vi "run pivot files.vi"() -> ()   [LabVIEW 2013]
uses:
  <vilib>/Utility/file.llb/Read From Spreadsheet File (DBL).vi
panel:
  in  "Tab Control":enum32{"Load Files", "Run"}(tab)
  in  "file path":path=path "C:/Program Files/Labview/user.lib/ROSforLV_0.1/Devices/Baxter/NIST2/Circles (Nick)"
  out "filenames":string[](array[string])=["Pivot a25 s15 r370 n0_0.csv", "Pivot a25 s20 r370 n0_0.csv", "Pivot a25 s20 r370 n0_5.csv", "Pivot a25 s20 r370 n1_0.csv", "Pivot a25 s20 r370 n1_5.csv", "Pivot a25 s20 r370 n2_0.csv", "Pivot a25 s20 r370 n2_5.csv", "Pivot a25 s20 r370 n3_0.csv", "Pivot a25 s20 r370 n3_5.csv", "Pivot a25 s20 r370 n4_0.csv", "Pivot a25 s25 r370 n0_0.csv", "Pivot a25 s30 r370 n0_0.csv", "Pivot a25 s35 r370 n0_0.csv"]
  out "Loop":i32
  out "of":i32
  in  "Abort":bool
  in  "Cycles":i32
  out "Status":string[](array[string])=["Initializing"]
  # "Execute this tab first to see the avialable files.\nThen remove the undesired trajectories before running on the other tab."
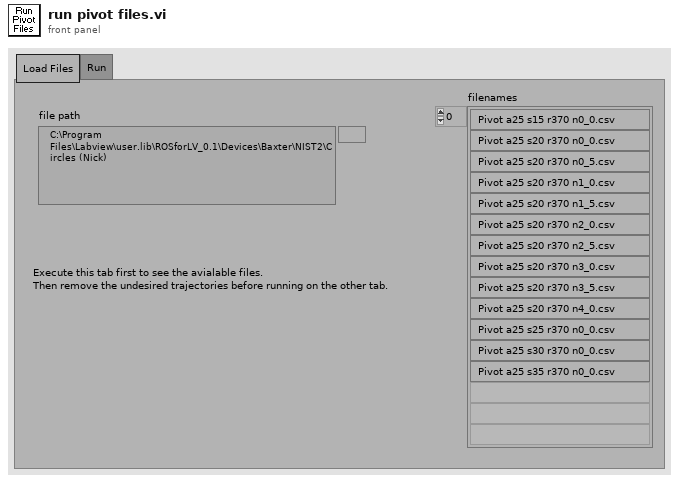
[diagram p1: front panel]
types:
  T1 = cluster{"cluster":cluster{"Name":string, "Joints":dbl[]}, "cluster":cluster{"Name":string, "Joints":dbl[]}}
  T2 = cluster{"cluster":cluster{"Name":string, "Joints":dbl[]}, "cluster":cluster{"Name":string, "Joints":dbl[]}}[]
  T3 = cluster{string, cluster{"cluster":cluster{"Name":string, "Joints":dbl[]}, "cluster":cluster{"Name":string, "Joints":dbl[]}}[]}
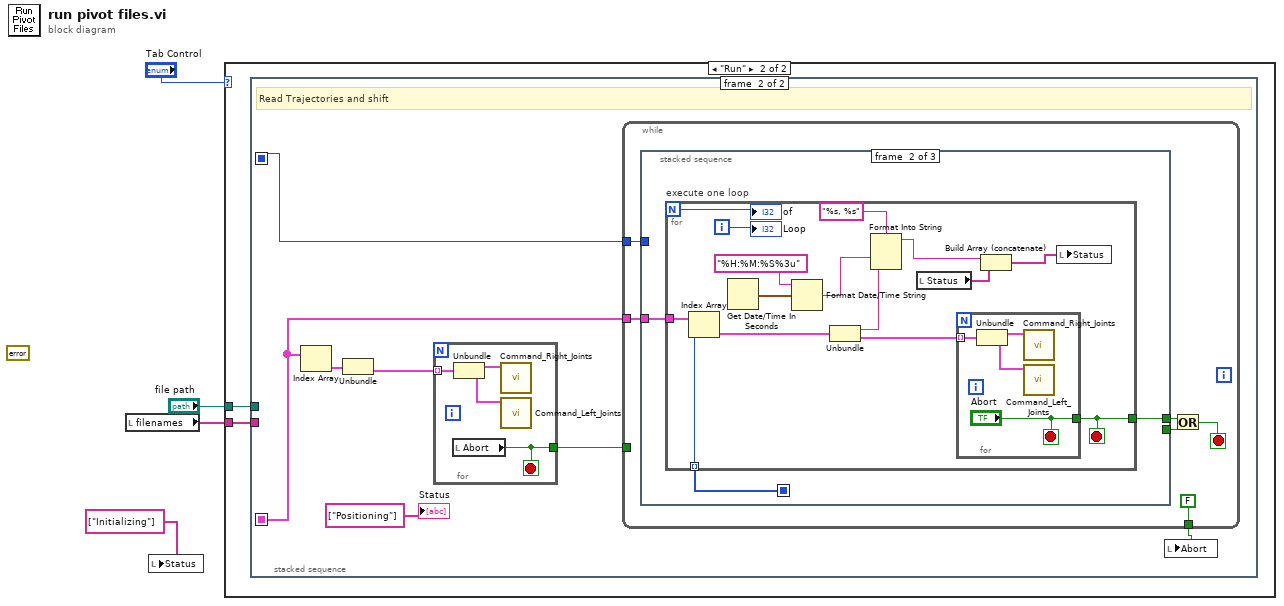
[diagram p0: block diagram]
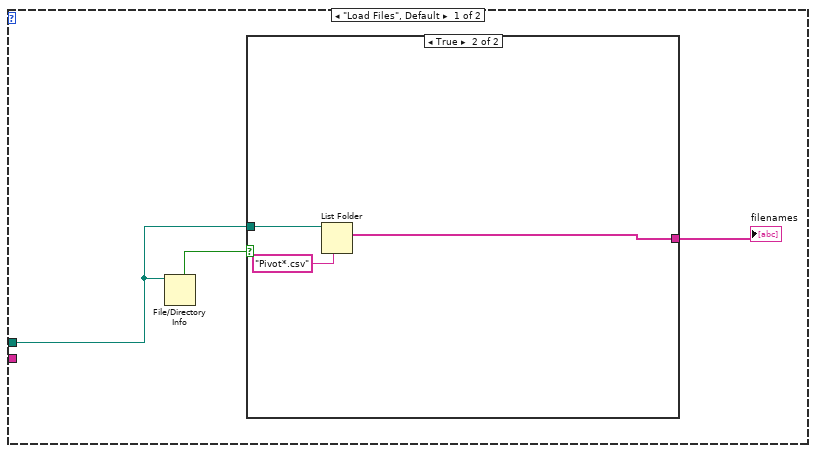
[diagram p2: hidden frame]
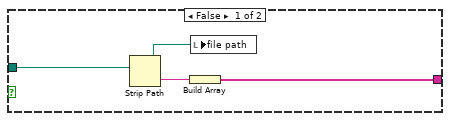
[diagram p3: hidden frame]
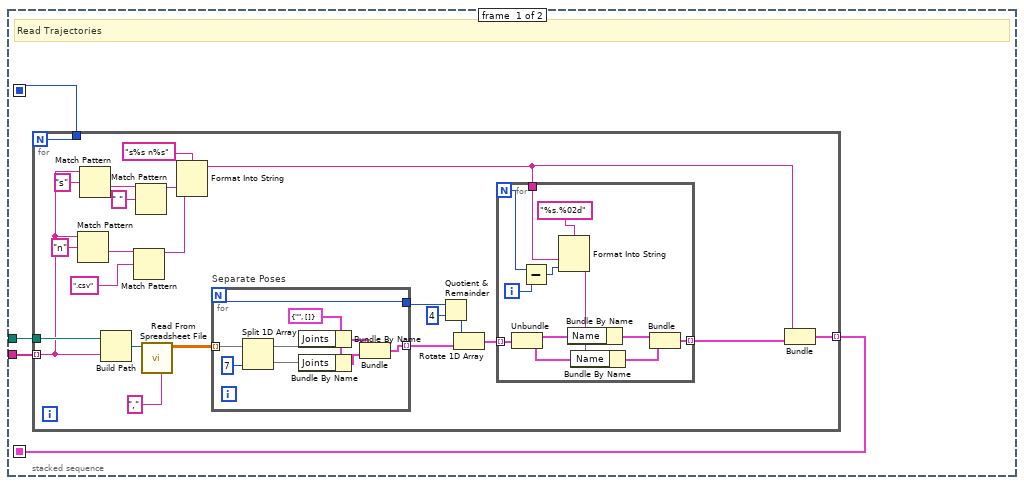
[diagram p4: hidden frame]
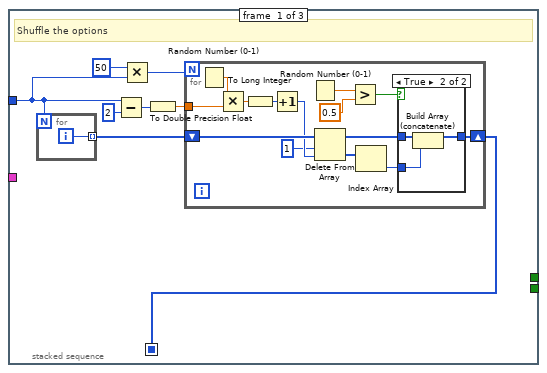
[diagram p5: hidden frame]
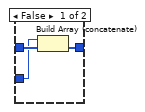
[diagram p6: hidden frame]
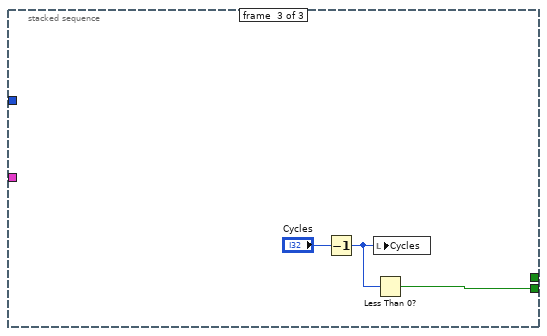
[diagram p7: hidden frame]
diagram:
  (unwired) errorcluster {"status"=FALSE, "code"=0, "source"=""} ("error out")
  n1 = local read "filenames"() -> (w2:string[])
  n2 = local write "Status"(string[] ["Initializing"]) -> ()
  n3 = case shown="\"Run\"" "Tab Control" {
    tunnel: "file path" -> [w5 w15]
    tunnel: w2 -> [_ w16]
    frame "Load Files", Default {
      n4 = File/Directory Info(path=w5) -> (directory=w7:bool)  [unwired: 1 in, 6 out]
      n5 = case shown="True" w7 {
        tunnel: w5 -> [w11 w14]
        tunnel: [w8 w12] -> w6
        frame False {
          n6 = Strip Path(path=w11) -> (stripped path=w10:path, name=w9:string)
          n7 = Build Array(w9) -> (w8:string[])
          n8 = local write "file path"(w10) -> ()
        }
        frame True {
          n9 = List Folder(path=w14, pattern="Pivot*.csv") -> (filenames=w12:string[])  [unwired: 2 in, 3 out]
        }
      }
      "filenames" <- w6
    }
    frame "Run" {
      n10 = stacked-sequence {
        seq-local: [w18 _] -> [_ w69]
        seq-local: [w17 _] -> [_ w71]
        tunnel: w16 -> [w20 _]
        tunnel: w15 -> [w19 _]
        frame #0 {
          # "Read Trajectories"
          n11 = for "Read Trajectories" {
            N -> [w22]
            tunnel: w20 -> [w28] mode=indexing
            tunnel: w19 -> [w43]
            tunnel: [w24] -> w18 mode=indexing
            tunnel: [w22] -> w17
            n12 = Match Pattern(string=w28, regular expression="n") -> (after substring=w30:string)  [unwired: 1 in, 3 out]
            n13 = Match Pattern(string=w28, regular expression="s") -> (after substring=w35:string)  [unwired: 1 in, 3 out]
            n14 = Build Path(base path=w43, name or relative path=w28) -> (appended path=w42:path)
            n15 = Match Pattern(string=w30, regular expression=".csv") -> (before substring=w27:string)  [unwired: 1 in, 3 out]
            n16 = Match Pattern(string=w35, regular expression=" ") -> (before substring=w33:string)  [unwired: 1 in, 3 out]
            n17 = call-poly <vilib>:"Read From Spreadsheet File.vi"("delimiter (\\t)"="," ("delimiter (\\t)"), "file path (dialog if empty)"=w42) -> ("all rows"=w40:dbl[][])  [unwired: 5 in, 4 out]
            n18 = Format Into String(format string="s%s n%s", w33, w27) -> (resulting string=w23:string)  [unwired: 2 in, 1 out]
            n19 = for "Separate Poses" {
              N -> [w56]
              tunnel: w40 -> [w64] mode=indexing
              tunnel: [w59] -> w37 mode=indexing
              tunnel: [w56] -> w21
              w60 = cluster{"Name":string, "Joints":dbl[]} {"Name"="", "Joints"=[]} ("cluster")
              n20 = Split 1D Array(array=w64, index=7) -> (first subarray=w62:dbl[], second subarray=w61:dbl[])
              n21 = Bundle By Name(cluster=w60, "Joints"=w62) -> (w58:cluster{"Name":string, "Joints":dbl[]})
              n22 = Bundle By Name(cluster=w60, "Joints"=w61) -> (w57:cluster{"Name":string, "Joints":dbl[]})
              n23 = Bundle("cluster"=w58, "cluster"=w57) -> (w59:T1)  [unwired: 1 in]
            }
            n24 = Quotient & Remainder(x=w21, y=4) -> (floor(x/y)=w39:i32)  [unwired: 1 out]
            n25 = Rotate 1D Array(1:w37, 2:w39) -> (0:w26:T2)
            n26 = for {
              N -> [w51]
              tunnel: w26 -> [w50] mode=indexing
              tunnel: [w44] -> w25 mode=indexing
              tunnel: w23 -> [w54]
              i -> [w53]
              n27 = Unbundle(w50) -> ("cluster"=w49:cluster{"Name":string, "Joints":dbl[]}, "cluster"=w48:cluster{"Name":string, "Joints":dbl[]})
              n28 = Subtract(x=w51, y=w53) -> (x-y=w52:i32)
              n29 = Format Into String(format string="%s.%02d", w54, w52) -> (resulting string=w47:string)  [unwired: 2 in, 1 out]
              n30 = Bundle By Name(cluster=w49, "Name"=w47) -> (w45:cluster{"Name":string, "Joints":dbl[]})
              n31 = Bundle By Name(cluster=w48, "Name"=w47) -> (w46:cluster{"Name":string, "Joints":dbl[]})
              n32 = Bundle("cluster"=w45, "cluster"=w46) -> (w44:T1)  [unwired: 1 in]
            }
            n33 = Bundle(w23, w25) -> (w24:T3)  [unwired: 1 in]
          }
        }
        frame #1 {
          # "Read Trajectories and shift"
          n34 = Index Array(array=w69) -> (element=w68:T3)  [unwired: 1 in]
          n35 = Unbundle(w68) -> (w67:T2)  [unwired: 1 out]
          n36 = for {
            tunnel: w67 -> [w75] mode=indexing
            tunnel: [w72] -> w65
            stop <- w72 stop-if-true
            n37 = local read "Abort"() -> (w72:bool)
            n38 = Unbundle(w75) -> ("cluster"=w74:cluster{"Name":string, "Joints":dbl[]}, "cluster"=w73:cluster{"Name":string, "Joints":dbl[]})
            n39 = call "Command_Right_Joints.vi"("Goal"=w74) -> ()  [unwired: 7 in, 2 out]
            n40 = call "Command_Left_Joints.vi"("Goal"=w73) -> ()  [unwired: 7 in, 2 out]
          }
          n41 = while {
            tunnel: w71 -> [w81]
            tunnel: w69 -> [w80]
            tunnel: [FALSE ("Abort")] -> w70
            tunnel: w65 -> [_]
            stop <- w77 stop-if-true
            n42 = stacked-sequence {
              seq-local: [w82 _ _] -> [_ w113 _]
              tunnel: w81 -> [w88 _ _]
              tunnel: w80 -> [_ w112 _]
              tunnel: [_ _ w133] -> w78
              tunnel: [_ w111 _] -> w79
              frame #0 {
                # "Shuffle the options"
                n43 = for {
                  N: w88 -> [_]
                  tunnel: [w110] -> w83 mode=indexing
                  i -> [w110]
                }
                n44 = Subtract(x=w88, y=2) -> (x-y=w86:i32)
                n45 = Multiply(x=50, y=w88) -> (x*y=w85:i32)
                n46 = To Double Precision Float(number=w86) -> (double precision float=w84:dbl)
                n47 = for {
                  N: w85 -> [_]
                  tunnel: w84 -> [w102]
                  shift-right: [w91] -> w82
                  shift-left: w83 -> [w99]
                  n48 = Random Number (0-1)() -> (number: 0 to 1=w103:dbl)
                  n49 = Multiply(x=w103, y=w102) -> (x*y=w101:dbl)
                  n50 = To Long Integer(number=w101) -> (32bit integer=w100:i32)
                  n51 = Increment(x=w100) -> (x+1=w98:i32)
                  n52 = Random Number (0-1)() -> (number: 0 to 1=w95:dbl)
                  n53 = Delete From Array(array=w99, length=1, index=w98) -> (deleted portion=w96:i32[], array with subset deleted=w92:i32[])
                  n54 = Greater?(x=w95, y=0.5) -> (0:w93:bool)
                  n55 = Index Array(array=w96) -> (element=w90:i32)  [unwired: 1 in]
                  n56 = case shown="True" w93 {
                    tunnel: w92 -> [w106 w109]
                    tunnel: [w105 w108] -> w91
                    tunnel: w90 -> [w104 w107]
                    frame False {
                      n57 = Build Array (concatenate)(w104, w106) -> (w105:i32[])
                    }
                    frame True {
                      n58 = Build Array (concatenate)(w109, w107) -> (w108:i32[])
                    }
                  }
                }
              }
              frame #1 {
                n59 = for "execute one loop" {
                  N -> [w122]
                  tunnel: w113 -> [w127] mode=indexing
                  tunnel: w112 -> [w128]
                  tunnel: [w120] -> w111
                  i -> [w123]
                  stop <- w120 stop-if-true
                  n60 = Index Array(array=w128, index=w127) -> (element=w126:T3)
                  n61 = Get Date/Time In Seconds() -> (seconds since 1Jan1904=w124:timestamp)
                  n62 = Format Date/Time String(time format string (%c)="%H:%M:%S%3u", seconds (now)=w124) -> (date/time string=w117:string)  [unwired: 1 in]
                  n63 = Unbundle(w126) -> (w118:string, w125:T2)
                  n64 = Format Into String(format string="%s, %s", w117, w118) -> (resulting string=w116:string)  [unwired: 2 in, 1 out]
                  n65 = local read "Status"() -> (w114:string[])
                  n66 = for {
                    tunnel: w125 -> [w132] mode=indexing
                    tunnel: ["Abort"] -> w120
                    stop <- "Abort" stop-if-true
                    n67 = Unbundle(w132) -> ("cluster"=w131:cluster{"Name":string, "Joints":dbl[]}, "cluster"=w130:cluster{"Name":string, "Joints":dbl[]})
                    n68 = call "Command_Right_Joints.vi"("Goal"=w131) -> ()  [unwired: 7 in, 2 out]
                    n69 = call "Command_Left_Joints.vi"("Goal"=w130) -> ()  [unwired: 7 in, 2 out]
                  }
                  n70 = Build Array (concatenate)(w116, w114) -> (w115:string[])
                  n71 = local write "Status"(w115) -> ()
                  "Loop" <- w123
                  "of" <- w122
                }
              }
              frame #2 {
                n72 = Decrement(x="Cycles") -> (x-1=w134:i32)
                n73 = local write "Cycles"(w134) -> ()
                n74 = Less Than 0?(x=w134) -> (x < 0?=w133:bool)
              }
            }
            n75 = Or(x=w79, y=w78) -> (x .or. y?=w77:bool)
          }
          n76 = local write "Abort"(w70) -> ()
          "Status" <- string[] ["Positioning"]
        }
      }
    }
  }
